vi "Init.vi"(8 "error in (no error)":errorcluster, 10 "Name":string, 11 "Category":string) -> (0 "error out":errorcluster, 3 "GetProfileParameter out":refnum<class "GetProfileParameter.lvclass">)   [LabVIEW 2020, in "obs-websocket.lvlib" / "GetProfileParameter.lvclass"]
uses:
  GetProfileParameter.lvclass
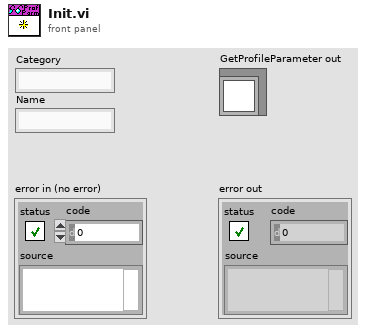
[diagram p1: front panel]
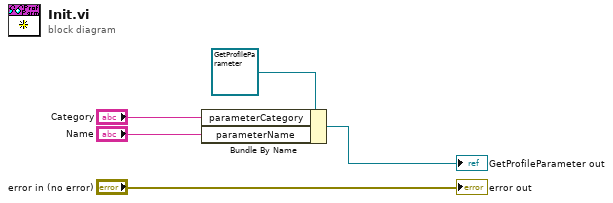
[diagram p0: block diagram]
diagram:
  n1 = Bundle By Name(cluster=refnum<class "GetProfileParameter.lvclass"> refnum ("GetProfileParameter in"), "parameterCategory"="Category", "parameterName"="Name") -> (→"GetProfileParameter out":refnum<class "GetProfileParameter.lvclass">)
  "error out" <- "error in (no error)"
